vi "RefreshEntireTree.vi"(7 "calling VI":refnum<vi>, 8 "error in":errorcluster, 10 "array":T1[](array[typedef]), 11 "tree ref":refnum<vi>) -> (0 "error out":errorcluster)   [LabVIEW 2025, in "CEF.lvlib"]
doc: "This VI refreshes the complete tree based on the node summary Copyright 2017 National Instruments Corporation\n\nLicensed under the Apache License, Version 2.0 (the \"License\"); you may not use this file except in compliance with the License. You may obtain a copy of the License at http://www.apache.org/licenses/LICENSE-2.0\nUnless required by applicable law or agreed to in writing, software distributed under the License is distributed on an \"AS IS\" BASIS, WITHOUT WARRANTIES OR CONDITIONS OF ANY KIND, either express or implied. See the License for the specific language governing permissions and limitations under the License."
uses:
  CEF.lvlib
  Node/Summary.ctl
  Node/CEF_Node.lvclass
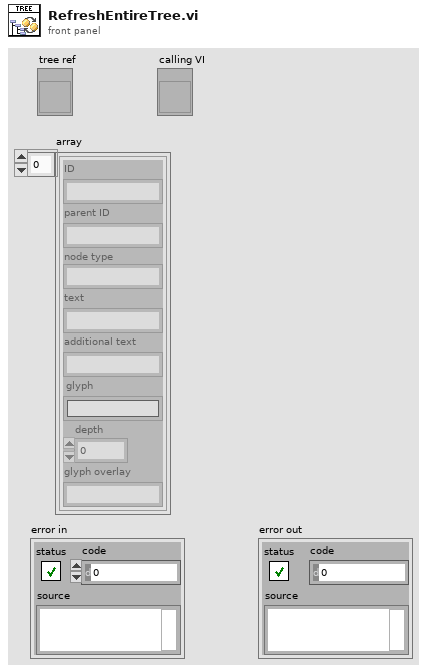
[diagram p1: front panel]
types:
  T1 = typedef "CEF.lvlib/CEF_Node.lvclass/Summary.ctl" = cluster{"ID":string, "parent ID":string, "node type":string, "text":string, "additional text":string, "glyph":string, "depth":i32, "glyph overlay":string}
  T2 = cluster{"Left Cell String":string, "Child text":string[], "Child Tag":string, "Item Indent":i32, "Child Only?":bool, "glyph Index":i32}
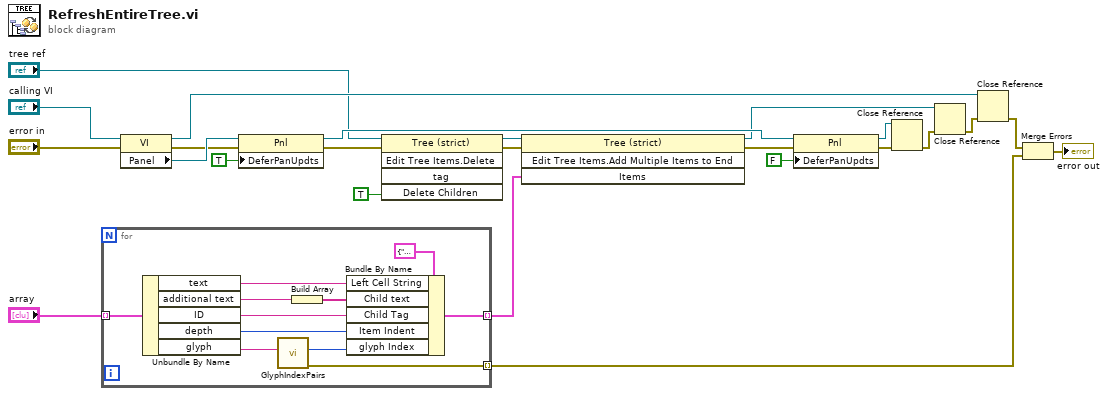
[diagram p0: block diagram]
diagram:
  n1 = for {
    tunnel: "array" -> [w35] mode=indexing
    tunnel: [w33] -> w8 mode=indexing
    tunnel: [w25] -> w3 mode=indexing
    n2 = Unbundle By Name(w35) -> ("text"=w32:string, "additional text"=w30:string, "ID"=w29:string, "depth"=w28:i32, "glyph"=w27:string)
    n3 = call "GlyphIndexPairs.vi"("glyph"=w27) -> ("error out"=w25:errorcluster, "index"=w26:i32)  [unwired: 9 in]
    n4 = Build Array(w30) -> (w31:string[])
    n5 = Bundle By Name(cluster=T2 {"Left Cell String"="", "Child text"=[], "Child Tag"="", "Item Indent"=0, "Child Only?"=FALSE, "glyph Index"=0} ("Item"), "Left Cell String"=w32, "Child text"=w31, "Child Tag"=w29, "Item Indent"=w28, "glyph Index"=w26) -> (w33:T2)
  }
  n6 = property class="VI"(reference="calling VI", error in="error in") -> (reference out=w15:refnum<vi>, error out=w22:errorcluster, "Panel"=w23:refnum<vi>)
  n7 = property class="Pnl"(reference=w23, error in=w22, "DeferPanUpdts"=TRUE ("Defer Panel Updates")) -> (reference out=w18:refnum<vi>, error out=w9:errorcluster)
  n8 = invoke class="Tree (strict)" method="Edit Tree Items.Delete"(reference="tree ref", error in=w9, "Delete Children"=TRUE ("Delete Children?")) -> (reference out=w10:refnum<vi>, error out=w7:errorcluster)  [unwired: 2 in, 3 out]
  n9 = invoke class="Tree (strict)" method="Edit Tree Items.Add Multiple Items to End"(reference=w10, error in=w7, "Items"=w8) -> (reference out=w1:refnum<vi>, error out=w6:errorcluster)  [unwired: 1 in, 2 out]
  n10 = property class="Pnl"(reference=w18, error in=w6, "DeferPanUpdts"=FALSE ("Defer Panel Updates")) -> (reference out=w2:refnum<vi>, error out=w17:errorcluster)
  n11 = Close Reference(reference=w2, error in (no error)=w17) -> (error out=w16:errorcluster)
  n12 = Close Reference(reference=w1, error in (no error)=w16) -> (error out=w14:errorcluster)
  n13 = Close Reference(reference=w15, error in (no error)=w14) -> (error out=w4:errorcluster)
  n14 = Merge Errors(w4, w3) -> (→"error out":errorcluster)
